vi "Measurement-BI.vi"(2 "Ctl Refnum 2":refnum<vi>, 3 "Ctl Refnum":refnum<vi>, 8 "error in (no error)":errorcluster, 9 "Byte Stream File Refnum":refnum<file>, 10 "客户仪器地址":refnum<visa-resource-name>="USB0::0x0471::0x2826::QF71600867::INSTR", 11 "起始偏压":dbl[][](array[numeric])=[[-5.0, 5.0, 21.0], [5.0, -5.0, 21.0], [-5.0, 0.0, 10.0]]) -> (0 "error out":errorcluster, 1 "Array":string[][](array[string]))   [LabVIEW 2017]
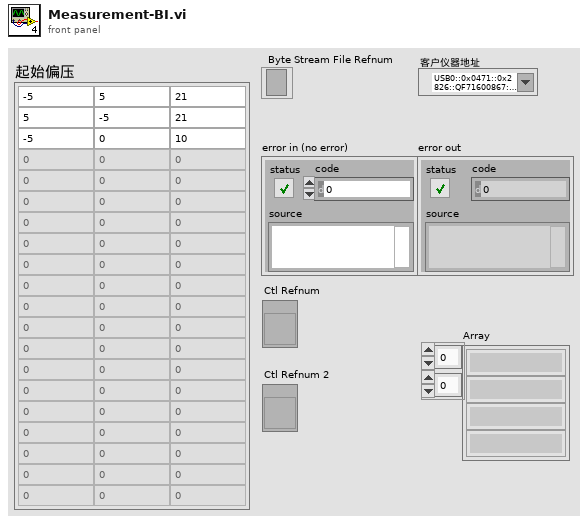
[diagram p1: front panel]
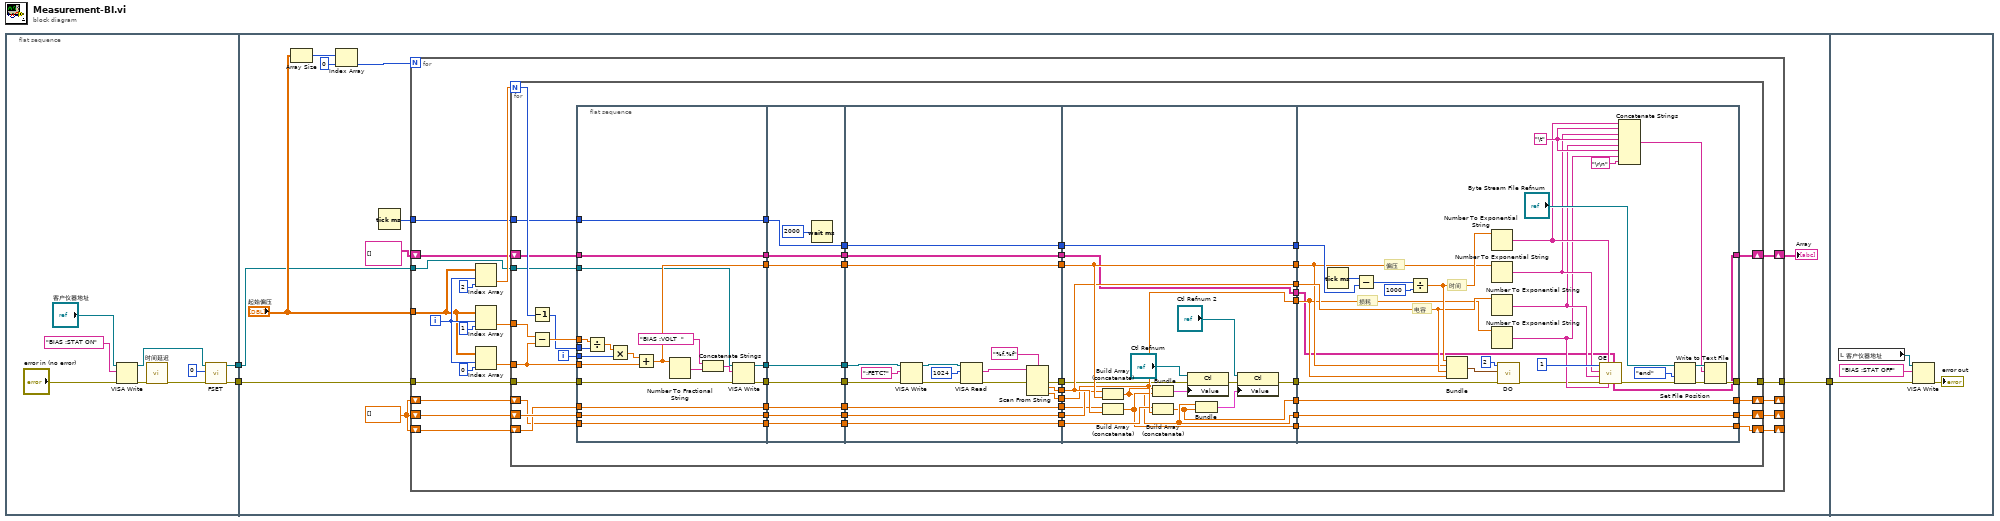
[diagram p0: block diagram]
diagram:
  n1 = flat-sequence {
    tunnel: [w7] -> w3
    tunnel: [w6] -> w2
    tunnel: w3 -> [w15]
    tunnel: w2 -> [w14]
    tunnel: [w13] -> w1
    tunnel: w1 -> [w192]
    frame #0 {
      n2 = VISA Write(VISA resource name="客户仪器地址", write buffer="BIAS :STAT ON" ("写入缓冲区"), error in (no error)="error in (no error)") -> (VISA resource name out=w8:refnum<visa-resource-name>, error out=w5:errorcluster)  [unwired: 1 out]
      n3 = call "时间延迟"("error in (no error)"=w5) -> ("error out"=w4:errorcluster)  [unwired: 10 in]
      n4 = call "FSET.vi"("error in (no error)"=w4, "Function (0: Cp-D)"=0, "VISA resource name"=w8) -> ("error out"=w6:errorcluster, "VISA resource name out"=w7:refnum<visa-resource-name>)  [unwired: 7 in]
    }
    frame #1 {
      w23 = dbl[] []
      n5 = Array Size(array="起始偏压") -> (size(s)=w21:i32[])
      n6 = Index Array(array=w21, index=0 ("索引")) -> (element=w19:i32)
      n7 = Tick Count (ms)() -> (millisecond timer value=w22:u32)
      n8 = for {
        N: w19 -> [_]
        shift-right: [w35] -> _
        shift-left: w23 -> [w36]
        shift-right: [w34] -> _
        shift-left: w23 -> [w33]
        shift-right: [w31] -> _
        shift-left: w23 -> [w32]
        tunnel: w22 -> [w30]
        tunnel: "起始偏压" -> [w29]
        shift-right: [w28] -> w16
        shift-left: string[][] [] -> [w27]
        tunnel: w15 -> [w26]
        tunnel: w14 -> [w25]
        tunnel: [w24] -> w13
        i -> [w40]
        n9 = Index Array(array=w29, index (row)=w40, index (col)=2 ("禁用的索引 (列)")) -> (element=w42:dbl)
        n10 = Index Array(array=w29, index (row)=w40, index (col)=1 ("禁用的索引 (列)")) -> (element=w38:dbl)
        n11 = Index Array(array=w29, index (row)=w40, index (col)=0 ("禁用的索引 (列)")) -> (element=w37:dbl)
        n12 = for {
          N: w42 -> [w93]
          tunnel: w38 -> [w95]
          tunnel: w37 -> [w90]
          shift-right: [w88] -> w35
          shift-left: w36 -> [w89]
          shift-right: [w84] -> w31
          shift-left: w32 -> [w85]
          shift-right: [w87] -> w34
          shift-left: w33 -> [w86]
          tunnel: w30 -> [w83]
          shift-right: [w54] -> w28
          shift-left: w27 -> [w50]
          tunnel: w26 -> [w48]
          tunnel: w25 -> [w47]
          tunnel: [w44] -> w24
          i -> [w91]
          n13 = Decrement(x=w93) -> (x-1=w92:i32)
          n14 = Subtract(x=w95, y=w90) -> (x-y=w94:dbl)
          n15 = flat-sequence {
            tunnel: w94 -> [w113]
            tunnel: w92 -> [w112]
            tunnel: w91 -> [w110]
            tunnel: w90 -> [w108]
            tunnel: w89 -> [w104]
            tunnel: [w104] -> w82
            tunnel: w86 -> [w103]
            tunnel: [w103] -> w81
            tunnel: w85 -> [w102]
            tunnel: [w102] -> w80
            tunnel: w83 -> [w101]
            tunnel: [w101] -> w79
            tunnel: [w105] -> w78
            tunnel: [w100] -> w57
            tunnel: [w99] -> w51
            tunnel: w50 -> [w99]
            tunnel: w48 -> [w98]
            tunnel: w47 -> [w97]
            tunnel: [w96] -> w45
            tunnel: w82 -> [w122]
            tunnel: [w122] -> w77
            tunnel: w81 -> [w121]
            tunnel: [w121] -> w76
            tunnel: w80 -> [w120]
            tunnel: [w120] -> w75
            tunnel: w79 -> [w119]
            tunnel: [w119] -> w74
            tunnel: w78 -> [w118]
            tunnel: [w118] -> w73
            tunnel: [w117] -> w58
            tunnel: w57 -> [w117]
            tunnel: [w116] -> w52
            tunnel: w51 -> [w116]
            tunnel: [w115] -> w46
            tunnel: w45 -> [w115]
            tunnel: w77 -> [w133]
            tunnel: [w133] -> w72
            tunnel: w76 -> [w132]
            tunnel: [w132] -> w71
            tunnel: w75 -> [w131]
            tunnel: [w131] -> w70
            tunnel: w74 -> [w130]
            tunnel: [w130] -> w69
            tunnel: [w135] -> w68
            tunnel: [w134] -> w67
            tunnel: w73 -> [w129]
            tunnel: [w129] -> w66
            tunnel: w58 -> [w128]
            tunnel: [w126] -> w55
            tunnel: [w125] -> w53
            tunnel: w52 -> [w125]
            tunnel: w46 -> [w124]
            tunnel: w72 -> [w156]
            tunnel: [w152] -> w65
            tunnel: [w153] -> w64
            tunnel: w71 -> [w155]
            tunnel: w70 -> [w154]
            tunnel: [w151] -> w63
            tunnel: w69 -> [w150]
            tunnel: [w150] -> w62
            tunnel: w68 -> [w158]
            tunnel: [w158] -> w61
            tunnel: w67 -> [w157]
            tunnel: [w157] -> w60
            tunnel: w66 -> [w159]
            tunnel: [w159] -> w59
            tunnel: [w144] -> w56
            tunnel: w55 -> [w145]
            tunnel: w53 -> [w149]
            tunnel: [w149] -> w49
            tunnel: [w180] -> w88
            tunnel: w65 -> [w180]
            tunnel: [w179] -> w87
            tunnel: w64 -> [w179]
            tunnel: [w178] -> w84
            tunnel: w63 -> [w178]
            tunnel: w62 -> [w189]
            tunnel: w61 -> [w175]
            tunnel: w60 -> [w173]
            tunnel: w59 -> [w174]
            tunnel: w56 -> [w161]
            tunnel: [w165] -> w54
            tunnel: w49 -> [w166]
            tunnel: [w172] -> w44
            frame #0 {
              n16 = Divide(x=w113, y=w112) -> (x/y=w111:dbl)
              n17 = Multiply(x=w111, y=w110) -> (x*y=w109:dbl)
              n18 = Add(x=w109, y=w108) -> (x+y=w105:dbl)
              n19 = Number To Fractional String(number=w105) -> (F-format string=w107:string)  [unwired: 3 in]
              n20 = Concatenate Strings("BIAS :VOLT  " ("字符串"), w107) -> (w106:string)
              n21 = VISA Write(VISA resource name=w98, write buffer=w106, error in (no error)=w97) -> (VISA resource name out=w96:refnum<visa-resource-name>, error out=w100:errorcluster)  [unwired: 1 out]
            }
            frame #1 {
              n22 = Wait (ms)(milliseconds to wait=u32 2000 ("等待时间（毫秒）")) -> ()  [unwired: 1 out]
            }
            frame #2 {
              n23 = VISA Write(VISA resource name=w124, write buffer=":FETC?" ("写入缓冲区"), error in (no error)=w128) -> (VISA resource name out=w139:refnum<visa-resource-name>, error out=w140:errorcluster)  [unwired: 1 out]
              n24 = VISA Read(VISA resource name=w139, byte count=u32 1024 ("字节总数"), error in (no error)=w140) -> (read buffer=w137:string, error out=w127:errorcluster)  [unwired: 2 out]
              n25 = Scan From String(format string="%f,%f" ("格式字符串"), input string=w137, error in=w127) -> (error out=w126:errorcluster, output 1=w135:dbl, output 2=w134:dbl)  [unwired: 3 in, 2 out]
            }
            frame #3 {
              n26 = Build Array (concatenate)(w156, w159) -> (w152:dbl[])
              n27 = Build Array (concatenate)(w155, w158) -> (w153:dbl[])
              n28 = Bundle(w152, w153) -> (w143:cluster{dbl[], dbl[]})  [unwired: 1 in]
              n29 = Build Array (concatenate)(w154, w157) -> (w151:dbl[])
              n30 = property class="Ctl"(reference="Ctl Refnum", error in=w145, "Value"=w143) -> (error out=w146:errorcluster)  [unwired: 1 out]
              n31 = Bundle(w152, w151) -> (w142:cluster{dbl[], dbl[]})  [unwired: 1 in]
              n32 = property class="Ctl"(reference="Ctl Refnum 2", error in=w146, "Value"=w142) -> (error out=w144:errorcluster)  [unwired: 1 out]
            }
            frame #4 {
              w183 = "\t"
              # "时间"
              # "损耗"
              # "电容"
              # "偏压"
              n33 = Tick Count (ms)() -> (millisecond timer value=w190:u32)
              n34 = Subtract(x=w190, y=w189) -> (x-y=w188:u32)
              n35 = Divide(x=w188, y=u32 1000) -> (x/y=w176:dbl)
              n36 = Bundle(w176, w174, w175, w173) -> (w163:cluster{dbl, dbl, dbl, dbl})  [unwired: 1 in]
              n37 = Number To Exponential String(number=w176) -> (E-format string=w170:string)  [unwired: 3 out]
              n38 = Number To Exponential String(number=w174) -> (E-format string=w169:string)  [unwired: 3 out]
              n39 = Number To Exponential String(number=w175) -> (E-format string=w168:string)  [unwired: 3 out]
              n40 = Number To Exponential String(number=w173) -> (E-format string=w167:string)  [unwired: 3 out]
              n41 = call "DO.vi"("error in (no error)"=w161, "数据输出"=w163, "功能编号"=2) -> ("error out"=w160:errorcluster)  [unwired: 8 in]
              n42 = call "OE.vi"("Array"=w166, "String 4"=w167, "String"=w170, "error in (no error)"=w160, "String 3"=w168, "String 2"=w169, "Numeric"=1) -> ("error out"=w164:errorcluster, "Array 2"=w165:string[][])  [unwired: 2 in, 1 out]
              n43 = Concatenate Strings(w170, w183, w169, w183, w168, w183, w167, "\r\n") -> (w185:string)
              n44 = Set File Position(refnum="Byte Stream File Refnum", from (0:start)=enum16{"start", "end", "current"}."end" ("自（0:起始）"), error in=w164) -> (refnum out=w186:refnum<file>, error out=w184:errorcluster)  [unwired: 1 out]
              n45 = Write to Text File(file (use dialog)=w186, text=w185, error in=w184) -> (error out=w172:errorcluster)  [unwired: 3 out]
            }
          }
        }
      }
      "Array" <- w16
    }
    frame #2 {
      n46 = local read "客户仪器地址"() -> (w193:refnum<visa-resource-name>)
      n47 = VISA Write(VISA resource name=w193, write buffer="BIAS :STAT OFF" ("写入缓冲区"), error in (no error)=w192) -> (error out=→"error out":errorcluster)  [unwired: 2 out]
    }
  }
